vi "Fix LV Timestamp String.vi"(1 "LabVIEW format string":string="2023-04-21T17:44:58.899-07:00:00") -> (0 "iso 8601 format string":string="2023-04-21T17:44:58.899-07:00")   [LabVIEW 2021, in "Logging.lvlib"]
doc: "Correct the LabVIEW-formatted time string to comply with ISO 8601 rules."
uses:
  Logging.lvlib
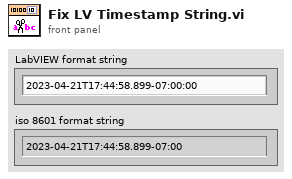
[diagram p1: front panel]
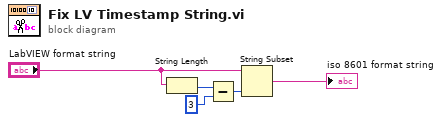
[diagram p0: block diagram]
diagram:
  n1 = String Length(string="LabVIEW format string") -> (length=w4:i32)
  n2 = Subtract(x=w4, y=3) -> (x-y=w5:i32)
  n3 = String Subset(string="LabVIEW format string", length (rest)=w5) -> (substring=→"iso 8601 format string":string)  [unwired: 1 in]
